vi "ColorSensor.vi"(0 "TestIndex":i32, 1 "通道":u8=1, 2 "地址":u8=1, 5 "等待时间（毫秒）":u32, 7 "功能选择":enum16{"读单独通道颜色值", "读单独通道光电值", "读全部光电值", "设置地址"}(ring)=enum."读全部光电值", 9 "延时":u32=150, 11 "error in (no error)":errorcluster caption="错误输入（无错误）", 12 "OnlyRead":bool, 13 "OnlyWrite":bool) -> (4 "返回结果":bool=TRUE, 6 "read buffer":string, 8 "数值数组":i32[](array[numeric]), 15 "error out":errorcluster={"status"=FALSE, "code"=1073676294, "source"="ColorSensor.vi中的VISA读取"} caption="错误输出")   [LabVIEW 2015]
uses:
  <vilib>/Instr/_visa.llb/VISA Configure Serial Port (Instr).vi
panel:
  out "发送的指令":string="3GET_ALL_LUX\r\n"
  out "VISA资源名称输出":refnum<visa-resource-name>="COM5"
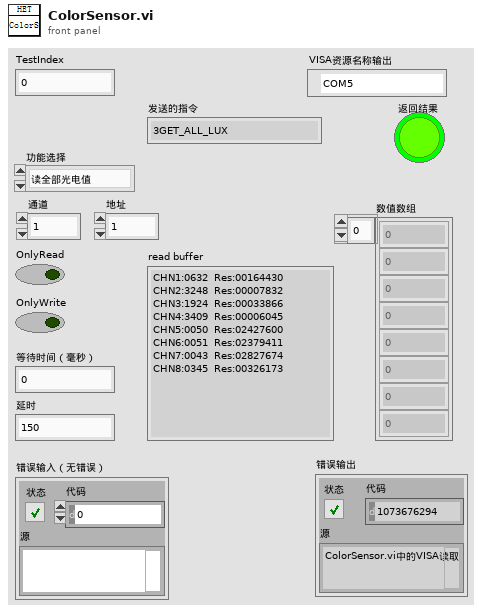
[diagram p1: front panel]
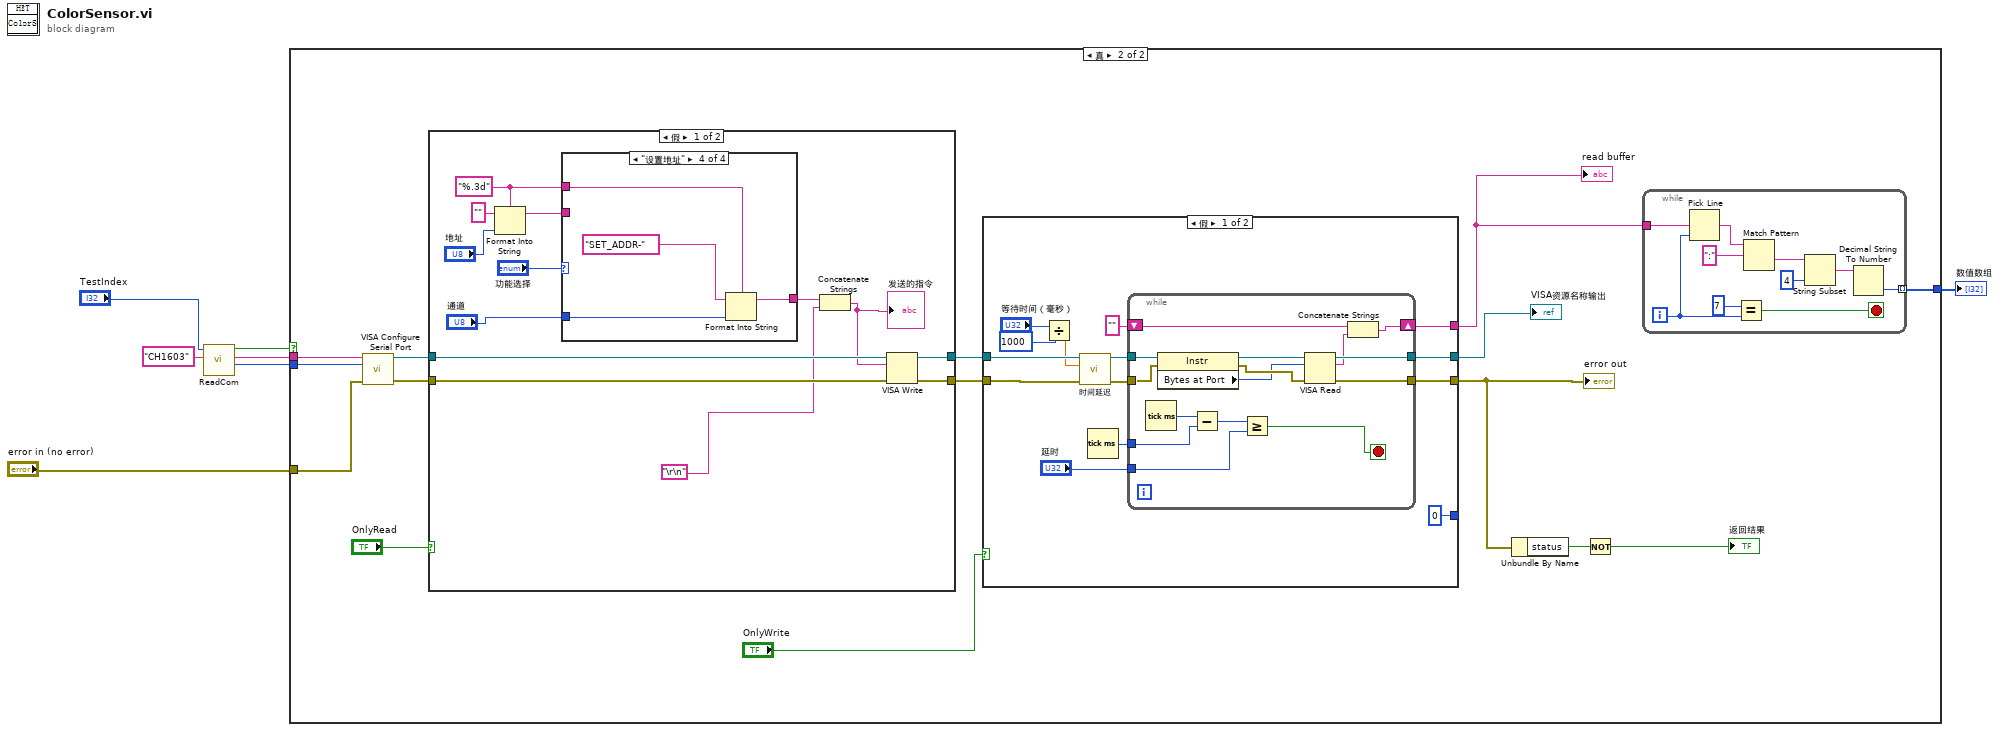
[diagram p0: block diagram]
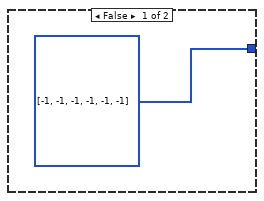
[diagram p2: hidden frame]
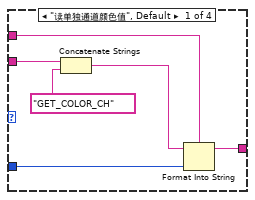
[diagram p3: hidden frame]
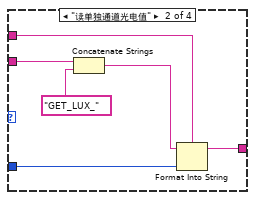
[diagram p4: hidden frame]
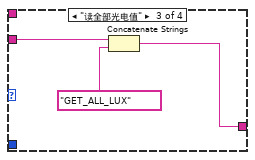
[diagram p5: hidden frame]
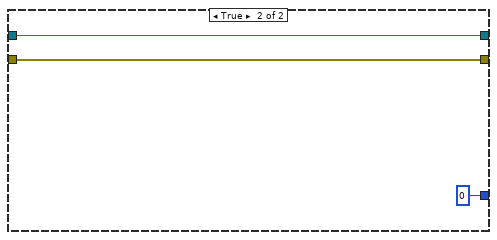
[diagram p7: hidden frame]
diagram:
  n1 = call "ReadCom.vi"("仪器名称"="CH1603", "MyIndex"="TestIndex") -> ("Baudrate"=w2:i32, "COM"=w3:string, "OK?"=w1:bool)  [unwired: 7 in]
  n2 = case shown="真" w1 {
    tunnel: "error in (no error)" -> [_ w17]
    tunnel: [i32[] [-1, -1, -1, -1, -1, -1] w13] -> w6
    tunnel: w3 -> [_ w10]
    tunnel: w2 -> [_ w9]
    frame False {
    }
    frame True {
      n3 = call-poly "VISA Configure Serial Port"("VISA resource name"=w10, "baud rate (9600)"=w9, "error in (no error)"=w17) -> ("VISA resource name out"=w14:refnum<visa-resource-name>, "error out"=w15:errorcluster)  [unwired: 11 in]
      n4 = case shown="假" "OnlyRead" {
        tunnel: [w46 w66] -> w21
        tunnel: [w45 w67] -> w20
        tunnel: w15 -> [w44 w66]
        tunnel: w14 -> [w43 w67]
        frame False {
          w40 = "%.3d"
          n5 = Format Into String(format string=w40, initial string="" ("初始字符串"), "地址") -> (resulting string=w39:string)  [unwired: 1 in, 1 out]
          n6 = case shown="\"设置地址\"" "功能选择" {
            tunnel: [w50 w58 w59 w64] -> w38
            tunnel: "通道" -> [w51 w57 _ w65]
            tunnel: w40 -> [w52 w56 _ w63]
            tunnel: w39 -> [w49 w55 w61 _]
            frame "读单独通道颜色值", Default {
              n7 = Concatenate Strings(w49, "GET_COLOR_CH" ("read buffer")) -> (w48:string)
              n8 = Format Into String(format string=w52, initial string=w48, w51) -> (resulting string=w50:string)  [unwired: 1 in, 1 out]
            }
            frame "读单独通道光电值" {
              n9 = Concatenate Strings(w55, "GET_LUX_" ("read buffer")) -> (w54:string)
              n10 = Format Into String(format string=w56, initial string=w54, w57) -> (resulting string=w58:string)  [unwired: 1 in, 1 out]
            }
            frame "读全部光电值" {
              n11 = Concatenate Strings(w61, "GET_ALL_LUX" ("read buffer")) -> (w59:string)
            }
            frame "设置地址" {
              n12 = Format Into String(format string=w63, initial string="SET_ADDR-" ("read buffer"), w65) -> (resulting string=w64:string)  [unwired: 1 in, 1 out]
            }
          }
          n13 = Concatenate Strings(w38, "\r\n") -> (w37:string)
          "发送的指令" <- w37
          n14 = VISA Write(VISA resource name=w43, write buffer=w37, error in (no error)=w44) -> (VISA resource name out=w45:refnum<visa-resource-name>, error out=w46:errorcluster)  [unwired: 1 out]
        }
        frame True {
        }
      }
      n15 = case shown="假" "OnlyWrite" {
        tunnel: [w80 _] -> w12
        tunnel: [w76 w97] -> w11
        tunnel: [w75 w98] -> w22
        tunnel: w21 -> [w74 w97]
        tunnel: w20 -> [w72 w98]
        tunnel: [0 ("y") 0 ("y")] -> _
        frame False {
          n16 = Divide(x="等待时间（毫秒）", y=u32 1000) -> (x/y=w69:dbl)
          n17 = call "时间延迟"("error in (no error)"=w74, "Delay Time (s)"=w69) -> ("error out"=w73:errorcluster)  [unwired: 9 in]
          n18 = Tick Count (ms)() -> (millisecond timer value=w78:u32)
          n19 = while {
            tunnel: w72 -> [w93]
            tunnel: [w95] -> w75
            tunnel: w73 -> [w91]
            tunnel: [w94] -> w76
            shift-right: [w87] -> w80
            shift-left: "" ("read buffer") -> [w86]
            tunnel: w78 -> [w84]
            tunnel: "延时" -> [w81]
            stop <- w82 stop-if-true
            n20 = Tick Count (ms)() -> (millisecond timer value=w85:u32)
            n21 = property class="Instr"(reference=w93, error in=w91) -> (reference out=w92:refnum<visa-resource-name>, error out=w90:errorcluster, "Bytes at Port"=w89:u32)
            n22 = Subtract(x=w85, y=w84) -> (x-y=w83:u32)
            n23 = Greater Or Equal?(x=w83, y=w81) -> (x >= y?=w82:bool)
            n24 = VISA Read(VISA resource name=w92, byte count=w89, error in (no error)=w90) -> (VISA resource name out=w95:refnum<visa-resource-name>, read buffer=w88:string, error out=w94:errorcluster)  [unwired: 1 out]
            n25 = Concatenate Strings(w86, w88) -> (w87:string)
          }
        }
        frame True {
        }
      }
      "error out" <- w11
      "VISA资源名称输出" <- w22
      "read buffer" <- w12
      n26 = Unbundle By Name(w11) -> ("status"=w23:bool)
      n27 = Not(x=w23) -> (.not. x?=→"返回结果":bool)
      n28 = while {
        tunnel: [w25] -> w13 mode=indexing
        tunnel: w12 -> [w24]
        i -> [w33]
        stop <- w31 stop-if-true
        n29 = Pick Line(multi-line string=w24, line index=w33) -> (output string=w30:string)  [unwired: 1 in]
        n30 = Equal?(x=7, y=w33) -> (x = y?=w31:bool)
        n31 = Match Pattern(string=w30, regular expression=":" ("搜索字符串/字符(-)")) -> (after substring=w28:string)  [unwired: 1 in, 3 out]
        n32 = String Subset(string=w28, length (rest)=4 ("长度（剩余）")) -> (substring=w26:string)  [unwired: 1 in]
        n33 = Decimal String To Number(string=w26) -> (number=w25:i32)  [unwired: 2 in, 1 out]
      }
    }
  }
  "数值数组" <- w6
